vi "S2C_M2p5942_Proc_ManageCtrls.vi"(8 "Error In":errorcluster, 9 "CtlRef":refnum<vi>) -> (0 "Error Out":errorcluster)   [LabVIEW 2024]
uses:
  S2C_M2p5942_Proc_Globals.vi
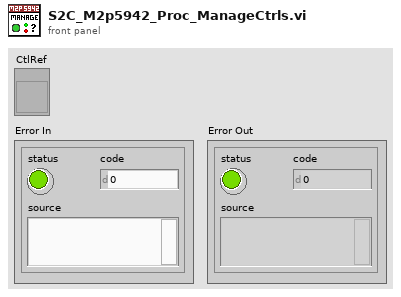
[diagram p1: front panel]
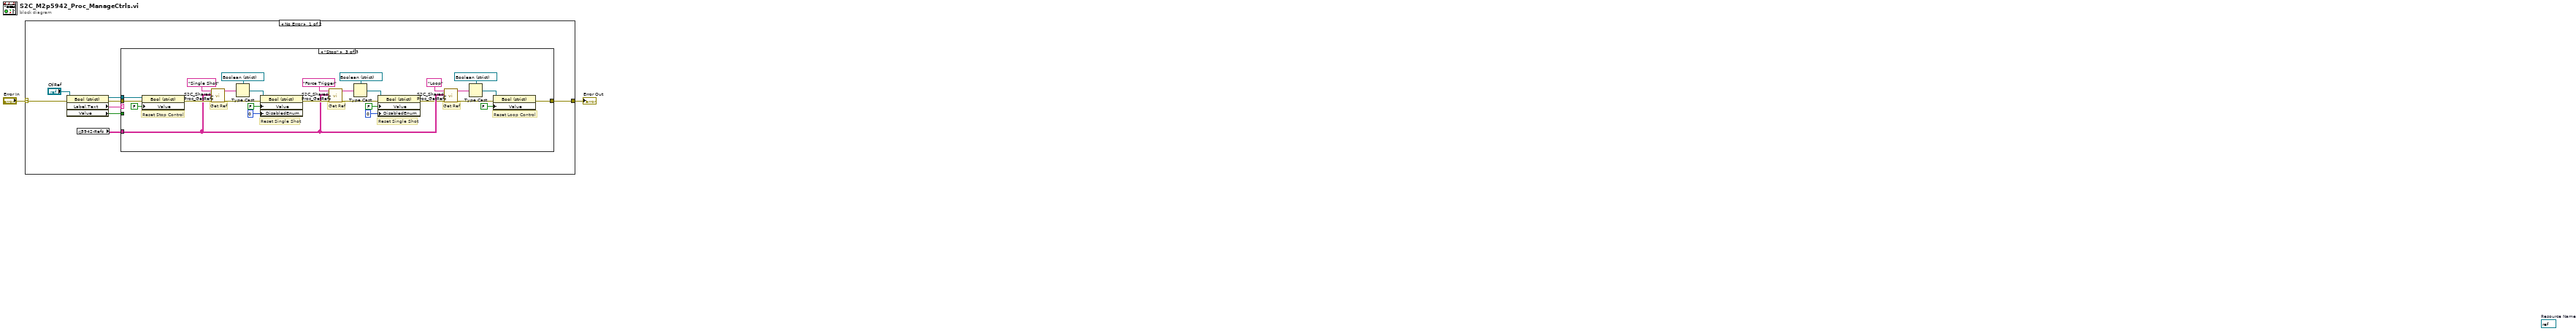
[diagram p0: block diagram]
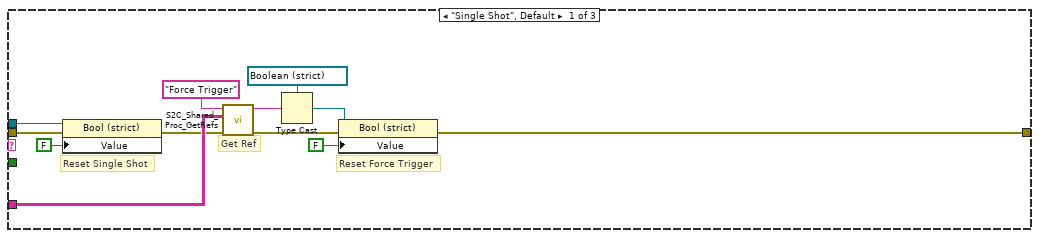
[diagram p2: hidden frame]
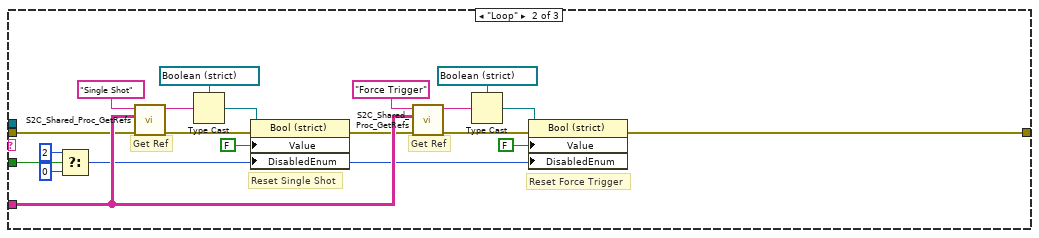
[diagram p3: hidden frame]
diagram:
  (unwired) refnum<visa-resource-name> refnum  # Resource Name
  n1 = case shown="No Error" "Error In" {
    selector: "Error In" -> [w3 w71]
    tunnel: [w4 w71] -> w2
    frame No Error {
      n2 = property class="Bool (strict)"(reference="CtlRef", error in=w3) -> (reference out=w6:refnum<vi>, error out=w8:errorcluster, "Label.Text"=w7:string, "Value"=w5:bool)
      n3 = global read "S2C_M2p5942_Proc_Globals.vi" "5942-Refs"() -> (w10:string[][])
      n4 = case shown="\"Stop\"" w7 {
        tunnel: w10 -> [w22 w42 w44]
        tunnel: [w11 w41 w53] -> w4
        tunnel: w8 -> [w14 w40 w57]
        tunnel: w6 -> [w13 _ w56]
        tunnel: w5 -> [_ w26 _]
        frame "Single Shot", Default {
          # "Reset Force Trigger"
          # "Get Ref"
          # "Reset Single Shot"
          n5 = property class="Bool (strict)"(reference=w13, error in=w14, "Value"=FALSE) -> (error out=w12:errorcluster)  [unwired: 1 out]
          n6 = call "S2C_Shared_Proc_GetRefs.vi"("Error In"=w12, "Refs"=w22, "Label"="Force Trigger") -> ("Error Out"=w20:errorcluster, "Reference"=w18:string)  [unwired: 7 in]
          n7 = Type Cast(type=refnum<vi> refnum ("Force Trigger?"), x=w18) -> (*(type *) &x=w19:refnum<vi>)
          n8 = property class="Bool (strict)"(reference=w19, error in=w20, "Value"=FALSE) -> (error out=w11:errorcluster)  [unwired: 1 out]
        }
        frame "Loop" {
          # "Reset Force Trigger"
          # "Get Ref"
          # "Reset Single Shot"
          # "Get Ref"
          n9 = Select(t=u8 2, s=w26, f=u8 0) -> (s? t:f=w23:u8)
          n10 = call "S2C_Shared_Proc_GetRefs.vi"("Error In"=w40, "Refs"=w42, "Label"="Single Shot") -> ("Error Out"=w34:errorcluster, "Reference"=w36:string)  [unwired: 7 in]
          n11 = Type Cast(type=refnum<vi> refnum ("Force Trigger?"), x=w36) -> (*(type *) &x=w35:refnum<vi>)
          n12 = property class="Bool (strict)"(reference=w35, error in=w34, "Value"=FALSE, "DisabledEnum"=w23) -> (error out=w27:errorcluster)  [unwired: 1 out]
          n13 = call "S2C_Shared_Proc_GetRefs.vi"("Error In"=w27, "Refs"=w42, "Label"="Force Trigger") -> ("Error Out"=w33:errorcluster, "Reference"=w31:string)  [unwired: 7 in]
          n14 = Type Cast(type=refnum<vi> refnum ("Force Trigger?"), x=w31) -> (*(type *) &x=w32:refnum<vi>)
          n15 = property class="Bool (strict)"(reference=w32, error in=w33, "Value"=FALSE, "DisabledEnum"=w23) -> (error out=w41:errorcluster)  [unwired: 1 out]
        }
        frame "Stop" {
          # "Reset Single Shot"
          # "Get Ref"
          # "Reset Stop Control"
          # "Reset Loop Control"
          # "Get Ref"
          # "Reset Single Shot"
          # "Get Ref"
          n16 = property class="Bool (strict)"(reference=w56, error in=w57, "Value"=FALSE) -> (error out=w54:errorcluster)  [unwired: 1 out]
          n17 = call "S2C_Shared_Proc_GetRefs.vi"("Error In"=w54, "Refs"=w44, "Label"="Single Shot") -> ("Error Out"=w65:errorcluster, "Reference"=w67:string)  [unwired: 7 in]
          n18 = Type Cast(type=refnum<vi> refnum ("Force Trigger?"), x=w67) -> (*(type *) &x=w66:refnum<vi>)
          n19 = property class="Bool (strict)"(reference=w66, error in=w65, "Value"=FALSE, "DisabledEnum"=u8 0) -> (error out=w45:errorcluster)  [unwired: 1 out]
          n20 = call "S2C_Shared_Proc_GetRefs.vi"("Error In"=w45, "Refs"=w44, "Label"="Force Trigger") -> ("Error Out"=w51:errorcluster, "Reference"=w49:string)  [unwired: 7 in]
          n21 = Type Cast(type=refnum<vi> refnum ("Force Trigger?"), x=w49) -> (*(type *) &x=w50:refnum<vi>)
          n22 = property class="Bool (strict)"(reference=w50, error in=w51, "Value"=FALSE, "DisabledEnum"=u8 0) -> (error out=w43:errorcluster)  [unwired: 1 out]
          n23 = call "S2C_Shared_Proc_GetRefs.vi"("Error In"=w43, "Refs"=w44, "Label"="Loop") -> ("Error Out"=w63:errorcluster, "Reference"=w61:string)  [unwired: 7 in]
          n24 = Type Cast(type=refnum<vi> refnum ("Force Trigger?"), x=w61) -> (*(type *) &x=w62:refnum<vi>)
          n25 = property class="Bool (strict)"(reference=w62, error in=w63, "Value"=FALSE) -> (error out=w53:errorcluster)  [unwired: 1 out]
        }
      }
    }
    frame Error {
    }
  }
  "Error Out" <- w2
